vi "Test OpenDeviceManager.vi"(8 "error in (no error)":errorcluster) -> (0 "error out":errorcluster)   [LabVIEW 2023]
uses:
  13421221-801b-4908-bf30-5190fb0063a2.vi
  <vilib>/addons/_JKI Toolkits/Caraya/classes/Assert/Assert False.vi
  <vilib>/addons/_JKI Toolkits/Caraya/classes/Assert/Assert Not Error.vi
  Classes/DeviceManager/DeviceManager.lvclass
  <vilib>/addons/_JKI Toolkits/Caraya/classes/Assert/Assert.lvclass
  <vilib>/addons/_JKI Toolkits/Caraya/classes/Test/Test.lvclass
panel:
  # "Connector Pane"
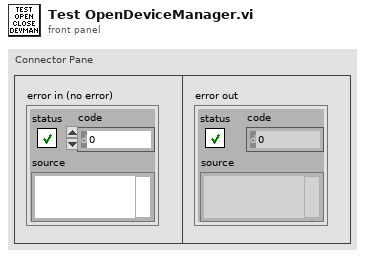
[diagram p1: front panel]
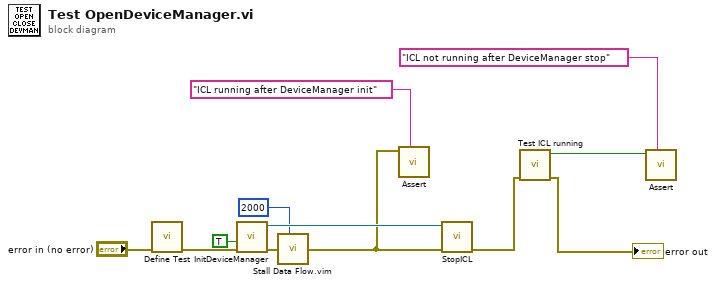
[diagram p0: block diagram]
diagram:
  n1 = call <vilib>:"Define Test.vi"("error in (no error)"="error in (no error)") -> ("error out"=w4:errorcluster)  [unwired: 9 in, 1 out]
  n2 = call "InitDeviceManager.vi"("error in (no error)"=w4, "start ICL on local host?"=TRUE) -> ("error out"=w11:errorcluster, "device manager"=w12:refnum<class "DeviceManager.lvclass">)  [unwired: 8 in]
  n3 = call "Stall Data Flow.vim"("value in"=w11, "milliseconds to wait"=u32 2000) -> ("value out"=w1:errorcluster)  [unwired: 1 out]
  n4 = call-poly <vilib>:"Assert.vi"("Label"="ICL running after DeviceManager init", "Not Error?"=w1) -> ()  [unwired: 8 in, 2 out]
  n5 = call-dynamic "StopICL.vi"("error in (no error)"=w1, "DeviceManager in"=w12) -> ("error out"=w9:errorcluster)  [unwired: 8 in, 1 out]
  n6 = call "Test ICL running.vi"("error in (no error)"=w9) -> ("error out"=→"error out":errorcluster, "icl.exe found"=w6:bool)  [unwired: 8 in, 1 out]
  n7 = call-poly <vilib>:"Assert.vi"("Label"="ICL not running after DeviceManager stop", "False?"=w6) -> ()  [unwired: 8 in, 2 out]
